vi "PD500 - Thermistors.vi"(8 "error in (no error)":errorcluster, 10 "Message IN":string) -> (0 "error out":errorcluster, 1 "Result (bool)":bool, 2 "Message OUT":string, 3 "Control Board OUT":refnum<visa-resource-name>, 5 "AUX Temps":dbl[](array[numeric]))   [LabVIEW 2022 SP3]
uses:
  Serial Board Com/Board Select.ctl
  Serial Board Com/ADCSelector BB.ctl
  Serial Board Com/ADCSelector GB.ctl
panel:
  in  "Board Selector":T1
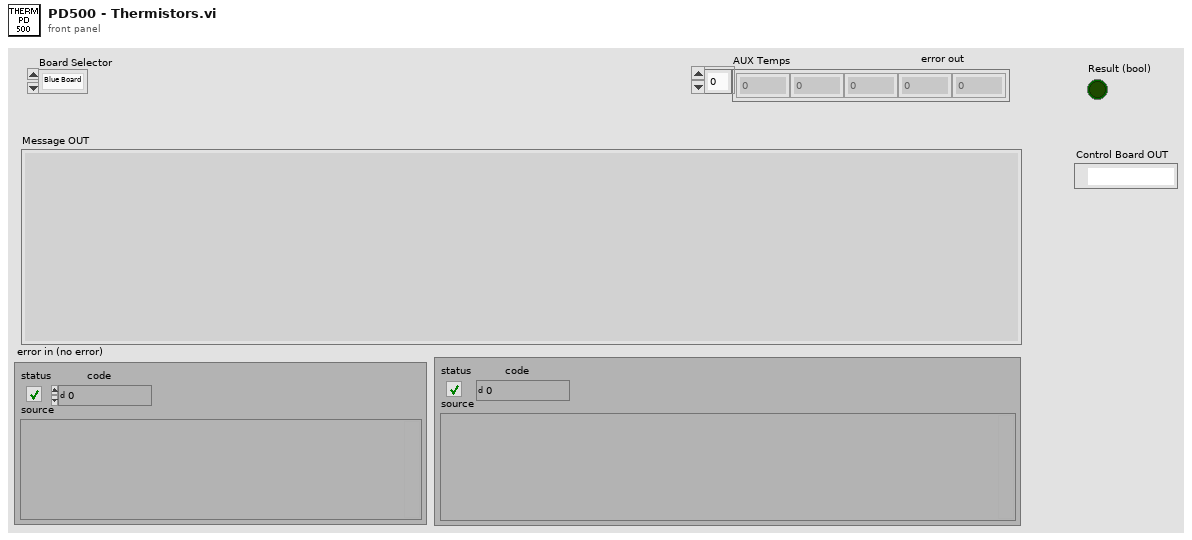
[diagram p1: front panel]
types:
  T1 = typedef "Board Select.ctl" = enum16{"Blue Board", "Green Board"}
  T2 = typedef "ADCSelector GB.ctl" = enum16{"INVA_ISENSE_U", "INVA_ISENSE_V", "INVA_ISENSE_W", "INVA_UDC", "INVA_TEMP", "HB_ISENSE", "AUX_ISENSE_U", "AUX_ISENSE_V", "AUX_ISENSE_W", "VLINE_AB", "VLINE_BC", "VLINE_CA", "REF_1P5V", "VSENSE_POS_24V", "VSENSE_POS_5V", "VSENSE_NEG_15V", "TEST_POINT", "INVB_ISENSE_U", "INVB_ISENSE_V", "INVB_ISENSE_W", "INVB_UDC", "INVB_TEMP", "HB_TEMP", "AUXA_TEMP", "AUXB_TEMP", "AUXC_TEMP", "VOUT_AB", "VOUT_BC", "VOUT_CA", "REF_2P5V", "VSENSE_POS_15V", "VSENSE_POS_3P3V", "NET_ANALYZER"}
  T3 = typedef "ADCSelector BB.ctl" = enum16{"INVA_ISENSE_U", "INVA_ISENSE_V", "INVA_ISENSE_W", "INVA_UDC", "INVA_TEMP", "HB_TEMP", "AUXB_TEMP", "VLINE_AB", "VLINE_BC", "VLINE_CA", "VSENSE_POS_24V", "VSENSE_POS_5V", "VSENSE_NEG_15V", "INVB_ISENSE_U", "INV_B_ISENSEV", "INVB_ISENSE_W", "INVB_UDC", "INVB_TEMP", "AUXA_TEMP", "AUXC_TEMP", "VOUT_AB", "VOUT_BC", "VOUT_CA", "VSENSE_POS_15V", "VSENSE_POS_3P3V", "TEST_POINT"}
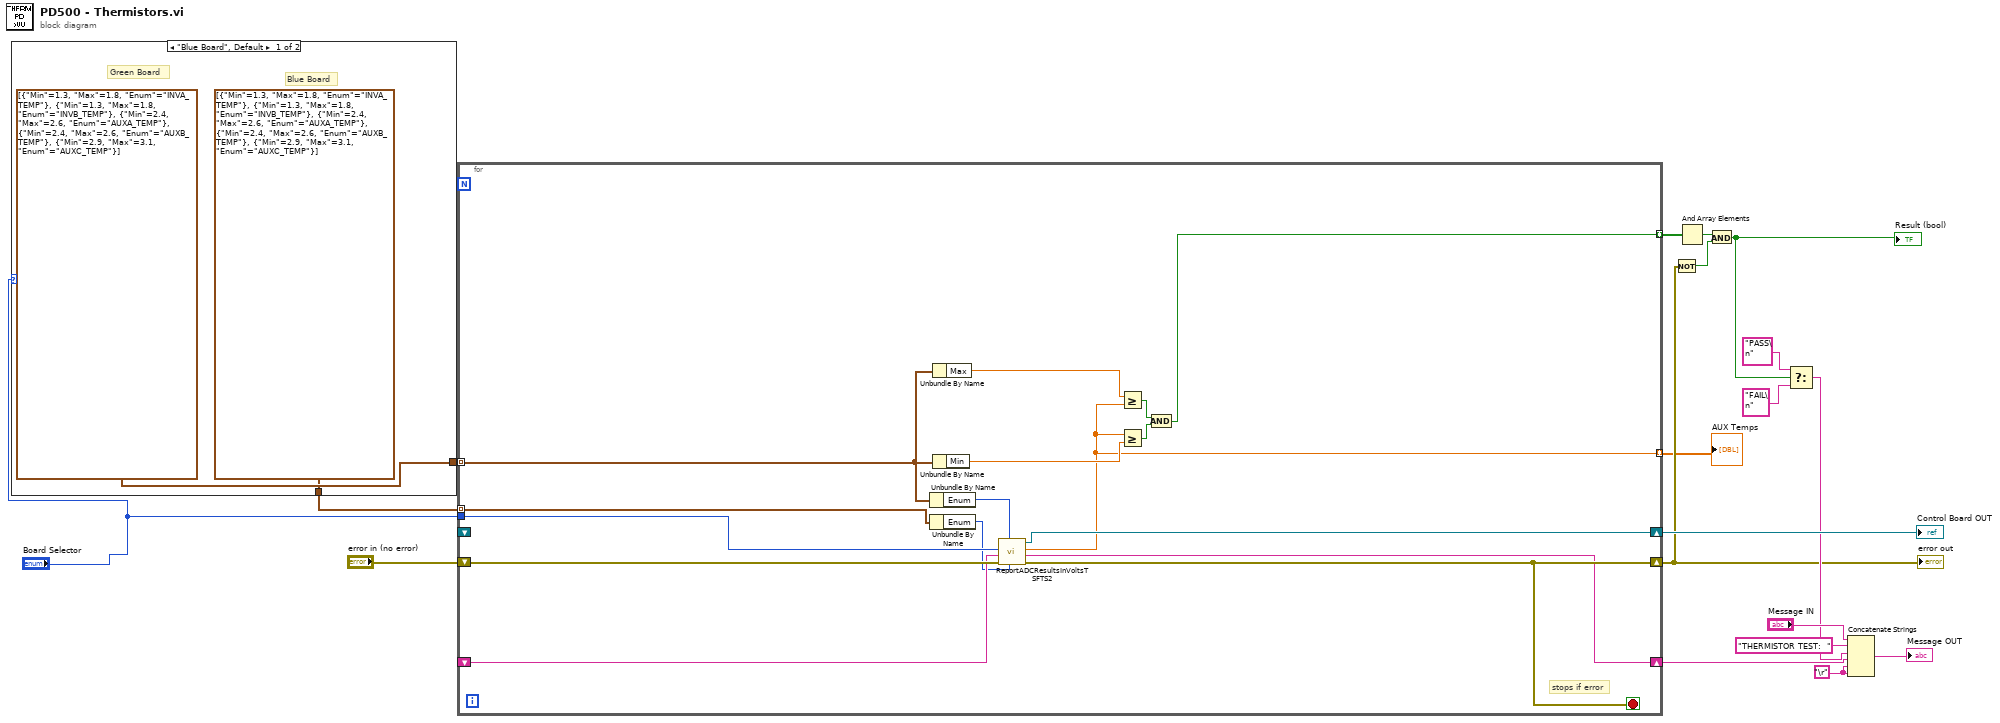
[diagram p0: block diagram]
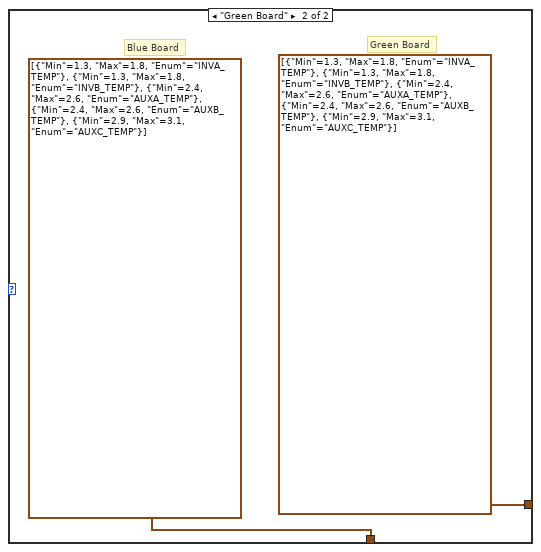
[diagram p2: hidden frame]
diagram:
  w10 = "\r"
  n1 = case shown="\"Blue Board\", Default" "Board Selector" {
    tunnel: [cluster{"Min":dbl, "Max":dbl, "Enum":T2}[] [{"Min"=1.3, "Max"=1.8, "Enum"=enum."INVA_TEMP"}, {"Min"=1.3, "Max"=1.8, "Enum"=enum."INVB_TEMP"}, {"Min"=2.4, "Max"=2.6, "Enum"=enum."AUXA_TEMP"}, {"Min"=2.4, "Max"=2.6, "Enum"=enum."AUXB_TEMP"}, {"Min"=2.9, "Max"=3.1, "Enum"=enum."AUXC_TEMP"}] cluster{"Min":dbl, "Max":dbl, "Enum":T2}[] [{"Min"=1.3, "Max"=1.8, "Enum"=enum."INVA_TEMP"}, {"Min"=1.3, "Max"=1.8, "Enum"=enum."INVB_TEMP"}, {"Min"=2.4, "Max"=2.6, "Enum"=enum."AUXA_TEMP"}, {"Min"=2.4, "Max"=2.6, "Enum"=enum."AUXB_TEMP"}, {"Min"=2.9, "Max"=3.1, "Enum"=enum."AUXC_TEMP"}]] -> w9
    tunnel: [cluster{"Min":dbl, "Max":dbl, "Enum":T3}[] [{"Min"=1.3, "Max"=1.8, "Enum"=enum."INVA_TEMP"}, {"Min"=1.3, "Max"=1.8, "Enum"=enum."INVB_TEMP"}, {"Min"=2.4, "Max"=2.6, "Enum"=enum."AUXA_TEMP"}, {"Min"=2.4, "Max"=2.6, "Enum"=enum."AUXB_TEMP"}, {"Min"=2.9, "Max"=3.1, "Enum"=enum."AUXC_TEMP"}] cluster{"Min":dbl, "Max":dbl, "Enum":T3}[] [{"Min"=1.3, "Max"=1.8, "Enum"=enum."INVA_TEMP"}, {"Min"=1.3, "Max"=1.8, "Enum"=enum."INVB_TEMP"}, {"Min"=2.4, "Max"=2.6, "Enum"=enum."AUXA_TEMP"}, {"Min"=2.4, "Max"=2.6, "Enum"=enum."AUXB_TEMP"}, {"Min"=2.9, "Max"=3.1, "Enum"=enum."AUXC_TEMP"}]] -> w3
    frame "Blue Board", Default {
      # "Blue Board"
      # "Green Board"
    }
    frame "Green Board" {
      # "Blue Board"
      # "Green Board"
    }
  }
  n2 = for {
    shift-right: [w39] -> w18
    shift-left: _ -> [_]
    shift-right: [w31] -> w4
    shift-left: "error in (no error)" -> [w38]
    tunnel: w9 -> [w34] mode=indexing
    tunnel: [w32] -> w8 mode=indexing
    shift-right: [w30] -> w11
    shift-left: _ -> [w29]
    tunnel: "Board Selector" -> [w28]
    tunnel: w3 -> [w26] mode=indexing
    tunnel: [w24] -> w1 mode=indexing
    stop <- w31 stop-if-true
    # "stops if error"
    n3 = Unbundle By Name(w34) -> ("Enum"=w27:T2)
    n4 = Unbundle By Name(w26) -> ("Enum"=w25:T3)
    n5 = Unbundle By Name(w34) -> ("Max"=w33:dbl)
    n6 = Unbundle By Name(w34) -> ("Min"=w35:dbl)
    n7 = call "ReportADCResultsInVoltsTSFTS2.vi"("Blue Board Enum"=w25, "Green Board Enum"=w27, "error in (no error)"=w38, "Message IN"=w29, "Board Selector"=w28) -> ("error out"=w31:errorcluster, "Message OUT"=w30:string, "Result"=w24:dbl, "VISA Refnum out"=w39:refnum<visa-resource-name>)  [unwired: 3 in]
    n8 = Greater Or Equal?(x=w33, y=w24) -> (x >= y?=w36:bool)
    n9 = Greater Or Equal?(x=w24, y=w35) -> (x >= y?=w37:bool)
    n10 = And(x=w36, y=w37) -> (x .and. y?=w32:bool)
  }
  "error out" <- w4
  "Control Board OUT" <- w18
  "AUX Temps" <- w1
  n11 = Not(x=w4) -> (.not. x?=w5:bool)
  n12 = And Array Elements(Boolean array=w8) -> (logical AND=w6:bool)
  n13 = And(x=w6, y=w5) -> (x .and. y?=w7:bool)
  "Result (bool)" <- w7
  n14 = Select(t="PASS\n", s=w7, f="FAIL\n") -> (s? t:f=w12:string)
  n15 = Concatenate Strings("Message IN", "THERMISTOR TEST:  " ("string"), w12, w11, w10, w10) -> (→"Message OUT":string)
